vi "Clear Comparator Bin.vi"   [LabVIEW 2017, in "Agilent E4980.lvlib"]
doc: "Limit table actions."
uses:
  Agilent E4980.lvlib
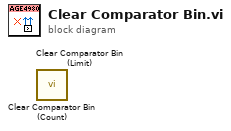
[diagram p0: block diagram]
diagram:
  n1 = call "Clear Comparator Bin (Count).vi"() -> ()  [unwired: 10 in, 2 out]
  n2 = call "Clear Comparator Bin (Limit).vi"() -> ()  [unwired: 10 in, 2 out]
